vi "Set new Sensitivity(SubVI).vi"(8 "error in (no error)":errorcluster, 9 "milliseconds to wait":u32=1000, 10 "Numeric":i32, 11 "Instrument parameters in":T1={"VISA Address"="", "GPIB/TCP Address"="", "String 1"="0_100", "String 2"="0", "Boolean 1"=FALSE, "Boolean 2"=FALSE, "Int 1"=0, "Int 2"=0, "Double 1"=0.0, "Double 2"=0.0}) -> (0 "error out":errorcluster, 2 "Sensitivity out":dbl, 3 "Instrument parameters out":T1)   [LabVIEW 2025]
uses:
  TYPE DEFS/S2DS_Instrument parameters.ctl
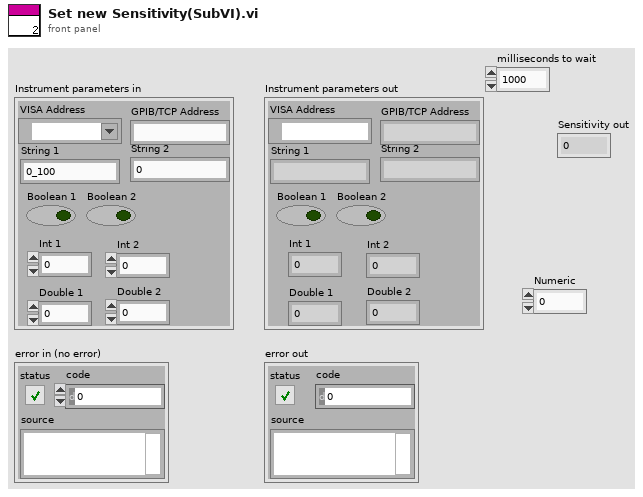
[diagram p1: front panel]
types:
  T1 = typedef "S2DS_Instrument parameters.ctl" = cluster{"VISA Address":refnum<visa-resource-name>, "GPIB/TCP Address":string, "String 1":string, "String 2":string, "Boolean 1":bool, "Boolean 2":bool, "Int 1":i32, "Int 2":i32, "Double 1":dbl, "Double 2":dbl}
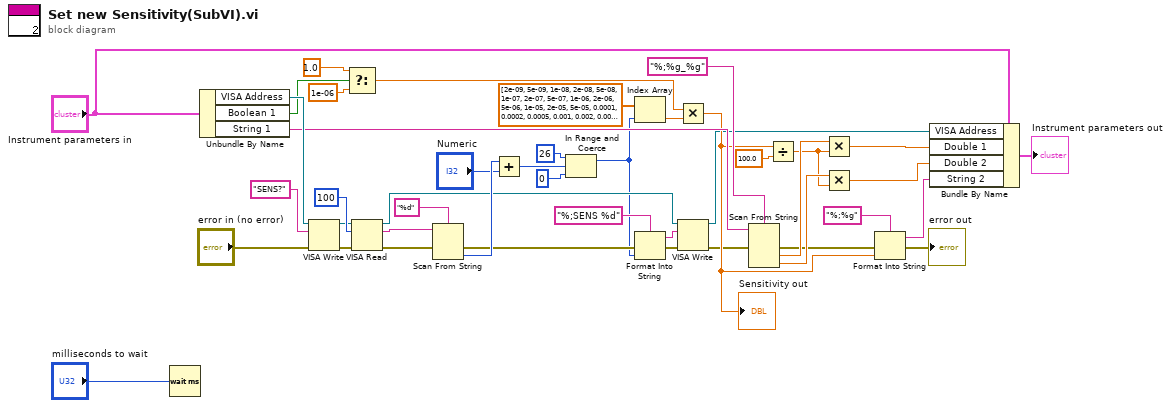
[diagram p0: block diagram]
diagram:
  n1 = Wait (ms)(milliseconds to wait="milliseconds to wait") -> ()  [unwired: 1 out]
  n2 = Unbundle By Name("Instrument parameters in") -> ("VISA Address"=w43:refnum<visa-resource-name>, "Boolean 1"=w31:bool, "String 1"=w42:string)
  n3 = VISA Write(VISA resource name=w43, write buffer="SENS?", error in (no error)="error in (no error)") -> (VISA resource name out=w23:refnum<visa-resource-name>, error out=w24:errorcluster)  [unwired: 1 out]
  n4 = Select(t=1.0, s=w31, f=1e-06) -> (s? t:f=w34:dbl)
  n5 = VISA Read(VISA resource name=w23, byte count=u32 100, error in (no error)=w24) -> (VISA resource name out=w10:refnum<visa-resource-name>, read buffer=w27:string, error out=w29:errorcluster)  [unwired: 1 out]
  n6 = Scan From String(format string="%d", input string=w27, error in=w29) -> (error out=w8:errorcluster, output 1=w14:i32)  [unwired: 2 in, 2 out]
  n7 = Add(x=w14, y="Numeric") -> (x+y=w5:i32)
  n8 = In Range and Coerce(upper limit=26, x=w5, lower limit=0) -> (coerced(x)=w2:i32)  [unwired: 1 out]
  n9 = Index Array(array=dbl[] [2e-09, 5e-09, 1e-08, 2e-08, 5e-08, 1e-07, 2e-07, 5e-07, 1e-06, 2e-06, 5e-06, 1e-05, 2e-05, 5e-05, 0.0001, 0.0002, 0.0005, 0.001, 0.002, 0.005, 0.01, 0.02, 0.05, 0.1, 0.2, 0.5, 1.0], index=w2) -> (element=w35:dbl)
  n10 = Format Into String(format string="%;SENS %d", error in=w8, w2) -> (resulting string=w11:string, error out=w9:errorcluster)  [unwired: 1 in]
  n11 = Multiply(x=w34, y=w35) -> (x*y=w19:dbl)
  "Sensitivity out" <- w19
  n12 = VISA Write(VISA resource name=w10, write buffer=w11, error in (no error)=w9) -> (VISA resource name out=w6:refnum<visa-resource-name>, error out=w7:errorcluster)  [unwired: 1 out]
  n13 = Scan From String(format string="%;%g_%g", input string=w42, error in=w7) -> (error out=w16:errorcluster, output 1=w37:dbl, output 2=w38:dbl)  [unwired: 3 in, 2 out]
  n14 = Divide(x=w19, y=100.0) -> (x/y=w20:dbl)
  n15 = Multiply(x=w37, y=w20) -> (x*y=w40:dbl)
  n16 = Multiply(x=w38, y=w20) -> (x*y=w41:dbl)
  n17 = Format Into String(format string="%;%g", error in=w16, w19) -> (resulting string=w17:string, error out=→"error out":errorcluster)  [unwired: 1 in]
  n18 = Bundle By Name(cluster="Instrument parameters in", "VISA Address"=w6, "Double 1"=w40, "Double 2"=w41, "String 2"=w17) -> (→"Instrument parameters out":T1)
